vi "Match.vi"(5 "Invert? [F]":bool, 7 "Regex? [F]":bool, 8 "error in (no error)":errorcluster, 10 "Label":string, 11 "MMI Scaling in":refnum<class "IObject.lvclass">) -> (0 "error out":errorcluster, 2 "Match?":bool, 3 "MMI Scaling out":refnum<class "IObject.lvclass">)   [LabVIEW 2013, in "IObject.lvclass"]
uses:
  IObject.lvclass
  IObject.lvclass/IObject.ctl
  <vilib>/regexp/Match Regular Expression.xnode
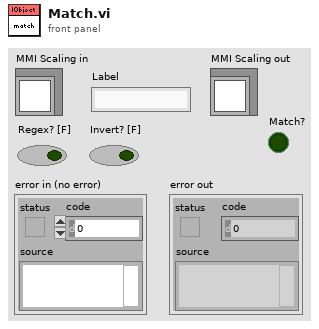
[diagram p1: front panel]
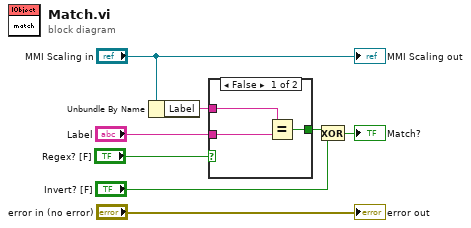
[diagram p0: block diagram]
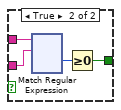
[diagram p2: hidden frame]
diagram:
  n1 = Unbundle By Name("MMI Scaling in") -> ("Label"=w5:string)
  n2 = case shown="False" "Regex? [F]" {
    tunnel: "Label" -> [w11 w14]
    tunnel: w5 -> [w10 w15]
    tunnel: [w9 w12] -> w4
    frame False {
      n3 = Equal?(x=w10, y=w11) -> (x = y?=w9:bool)
    }
    frame True {
      n4 = xnode "Match Regular Expression"("input string"=w15, "regular expression"=w14) -> ("offset past match"=w13:i32)  [unwired: 4 in, 4 out]
      n5 = Greater Or Equal To 0?(x=w13) -> (x >= 0?=w12:bool)
    }
  }
  n6 = Exclusive Or(1:"Invert? [F]", 2:w4) -> (0:→"Match?":bool)
  "error out" <- "error in (no error)"
  "MMI Scaling out" <- "MMI Scaling in"
